vi "Format Message String.vi"(9 "ID":string, 10 "Data":string, 11 "Command":string) -> (3 "Message":string)   [LabVIEW 2019, in "RemoteControl.lvlib" / "RemoteControl.lvclass"]
uses:
  RemoteControl.lvclass
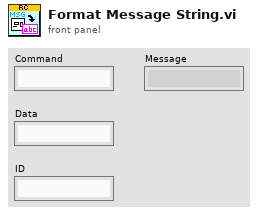
[diagram p1: front panel]
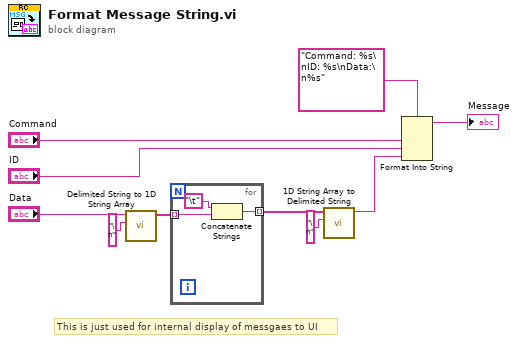
[diagram p0: block diagram]
diagram:
  # "This is just used for internal display of messgaes to UI"
  n1 = call <vilib>:"Delimited String to 1D String Array.vi"("delimiter"="\n", "delimited string"="Data") -> ("string array"=w9:string[])  [unwired: 9 in]
  n2 = for {
    tunnel: w9 -> [w13] mode=indexing
    tunnel: [w12] -> w8 mode=indexing
    n3 = Concatenate Strings("\t", w13) -> (w12:string)
  }
  n4 = call <vilib>:"1D String Array to Delimited String.vi"("delimiter"="\n", "string array"=w8) -> ("delimited string"=w4:string)  [unwired: 9 in]
  n5 = Format Into String(format string="Command: %s\nID: %s\nData:\n%s", "Command", "ID", w4) -> (resulting string=→"Message":string)  [unwired: 2 in, 1 out]
